vi "Edit_Raw_DF_Remote.vi"(4 "Edit Raw Data Header Info":bool, 5 "New Values In":string[](array[string])=["Test data5"], 6 "New Chs In":string[](array[string])=["30-10-03:New:Channel new5"], 7 "Current Filename":path) -> (0 "error out":errorcluster, 1 "Original values":string[](array[string]), 2 "File Not Changed?":bool, 3 "Filetype":string)   [LabVIEW 2010]
panel:
  in  "type specifier VI Refnum (for type only)":refnum<vi>
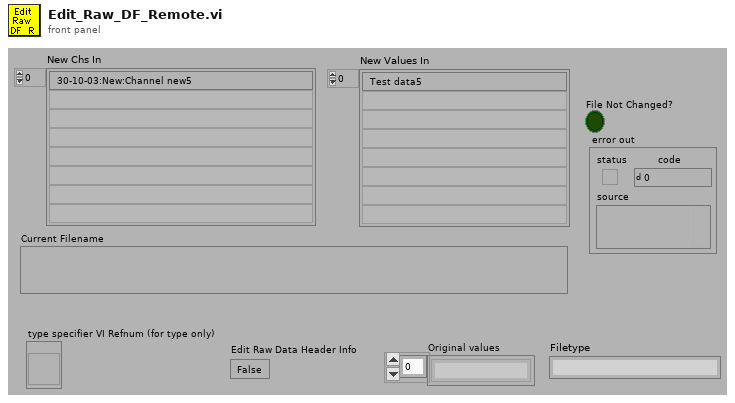
[diagram p1: front panel]
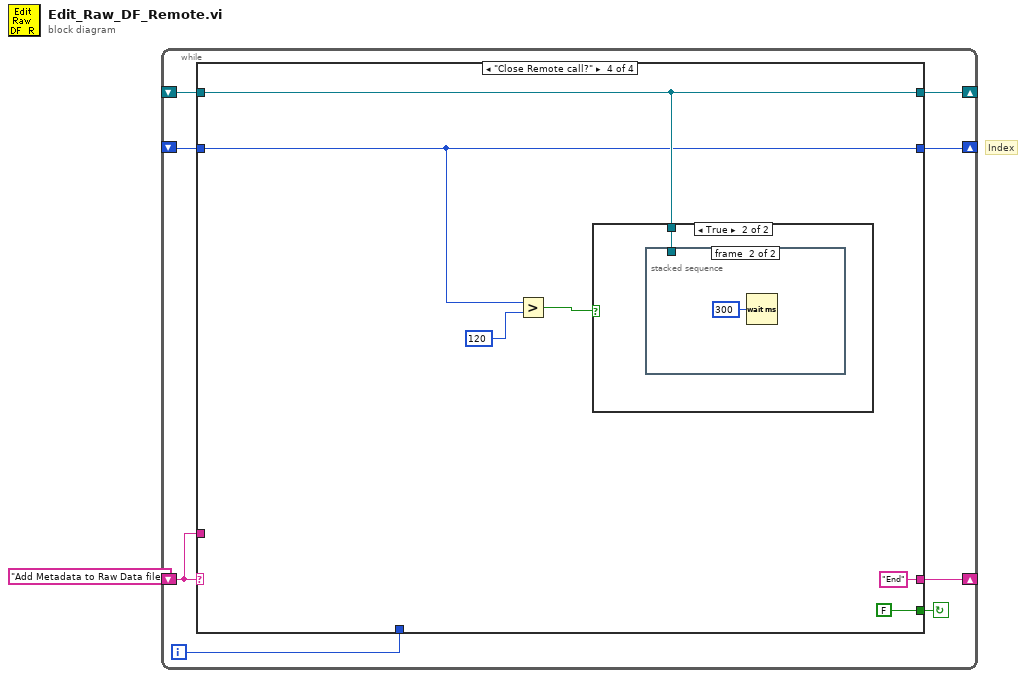
[diagram p0: block diagram]
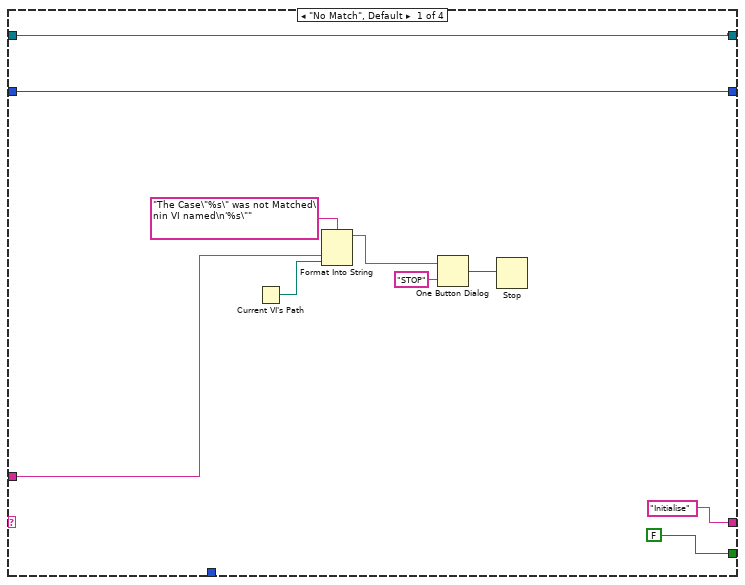
[diagram p2: hidden frame]
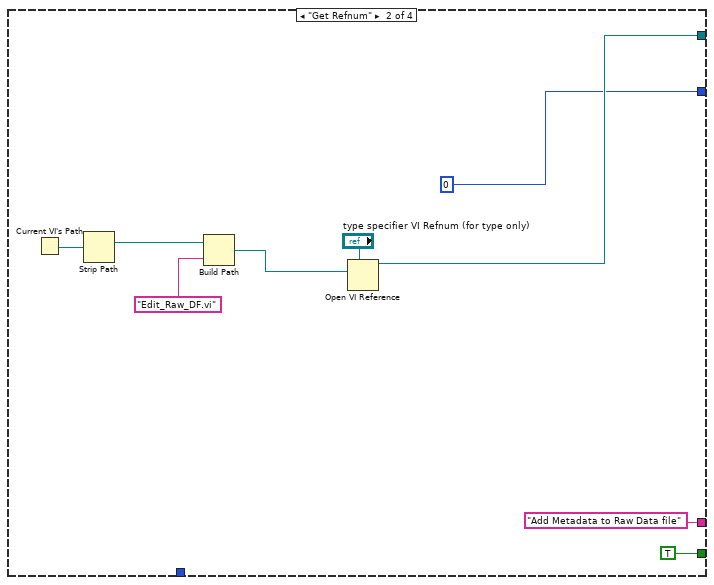
[diagram p3: hidden frame]
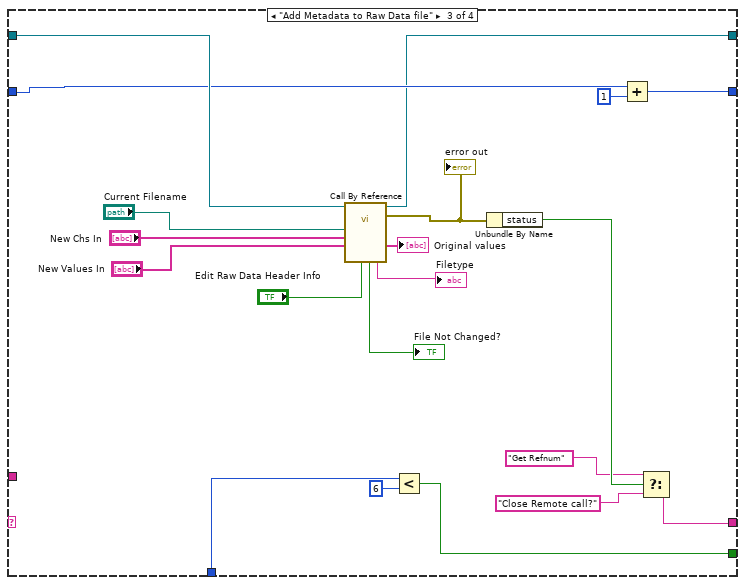
[diagram p4: hidden frame]
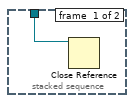
[diagram p6: hidden frame]
diagram:
  # "Index"
  n1 = while {
    shift-left: _ -> [w6]
    shift-right: [w7] -> _
    shift-left: "Add Metadata to Raw Data file" -> [w8]
    shift-right: [w9] -> _
    shift-right: [w4] -> _
    shift-left: _ -> [w3]
    i -> [w2]
    stop <- w5 continue-if-true
    n2 = case shown="\"Close Remote call?\"" w8 {
      tunnel: [FALSE TRUE w37 FALSE] -> w5
      tunnel: ["Initialise" "Add Metadata to Raw Data file" w45 "End"] -> w9
      tunnel: w8 -> [w14 _ _ _]
      tunnel: [w11 0 w40 w51] -> w7
      tunnel: w6 -> [w11 _ w42 w51]
      tunnel: [w10 w27 w31 w53] -> w4
      tunnel: w3 -> [w10 _ w47 w53]
      tunnel: w2 -> [_ _ w39 _]
      frame "No Match", Default {
        n3 = Current VI's Path() -> (path=w13:path)
        n4 = Format Into String(format string="The Case\"%s\" was not Matched\nin VI named\n'%s\"" ("Format String"), w14, w13) -> (resulting string=w17:string)  [unwired: 2 in, 1 out]
        n5 = One Button Dialog(message=w17, button name ("OK")="STOP") -> (true=w15:bool)
        n6 = Stop(stop? (T)=w15) -> ()
      }
      frame "Get Refnum" {
        n7 = Current VI's Path() -> (path=w23:path)
        n8 = Strip Path(path=w23) -> (stripped path=w22:path)  [unwired: 1 out]
        n9 = Build Path(base path=w22, name or relative path="Edit_Raw_DF.vi") -> (appended path=w20:path)
        n10 = Open VI Reference(type specifier VI Refnum (for type only)="type specifier VI Refnum (for type only)", vi path=w20) -> (vi reference=w27:refnum<vi>)  [unwired: 1 in, 4 out]
      }
      frame "Add Metadata to Raw Data file" {
        n11 = call-by-ref "?"(reference=w47, "Edit Raw Data Header Info"="Edit Raw Data Header Info", "New Values In"="New Values In", "New Chs In"="New Chs In", "Data filename"="Current Filename") -> (reference out=w31:refnum<vi>, error out=w48:errorcluster, "Filetype"=→"Filetype":string, "Original values"=→"Original values":string[], "File Not Changed?"=→"File Not Changed?":bool)  [unwired: 3 in, 1 out]
        "error out" <- w48
        n12 = Less?(x=w39, y=6) -> (x < y?=w37:bool)
        n13 = Unbundle By Name(w48) -> ("status"=w46:bool)
        n14 = Add(x=w42, y=1) -> (x+y=w40:i32)
        n15 = Select(t="Get Refnum", s=w46, f="Close Remote call?") -> (s? t:f=w45:string)
      }
      frame "Close Remote call?" {
        n16 = Greater?(x=w51, y=120) -> (0:w49:bool)
        n17 = case shown="True" w49 {
          tunnel: w53 -> [_ w55]
          frame False {
          }
          frame True {
            n18 = stacked-sequence {
              tunnel: w55 -> [w56 _]
              frame #0 {
                n19 = Close Reference(reference=w56) -> ()  [unwired: 1 in, 1 out]
              }
              frame #1 {
                n20 = Wait (ms)(milliseconds to wait=u32 300) -> ()  [unwired: 1 out]
              }
            }
          }
        }
      }
    }
  }
